vi "Check for Authorization.vi"(8 "error in":errorcluster, 10 "JSON":string, 11 "nats connection in":T1) -> (0 "error out":errorcluster, 2 "dup JSON":string, 3 "dup nats connection":T1)   [LabVIEW 2013, in "NATS Core.lvlib"]
doc: "Check if the server is requesting some form of authorization. If so, verify the client has provided some form of authorization regardless of validity."
uses:
  NATS Core.lvlib
  Controls/nats connection.ctl
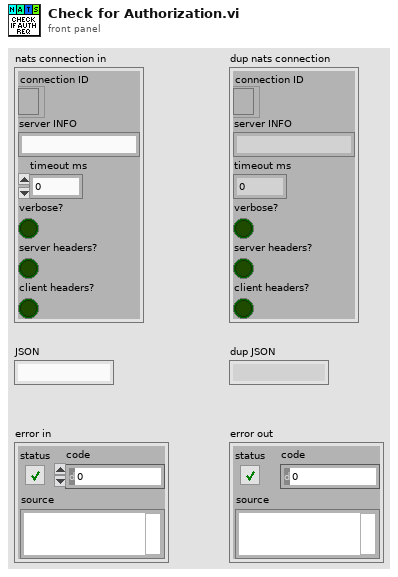
[diagram p1: front panel]
types:
  T1 = typedef "NATS Core.lvlib/nats connection.ctl" = cluster{"connection ID":refnum<k5>, "server INFO":string, "timeout ms":i32, "verbose?":bool, "server headers?":bool, "client headers?":bool}
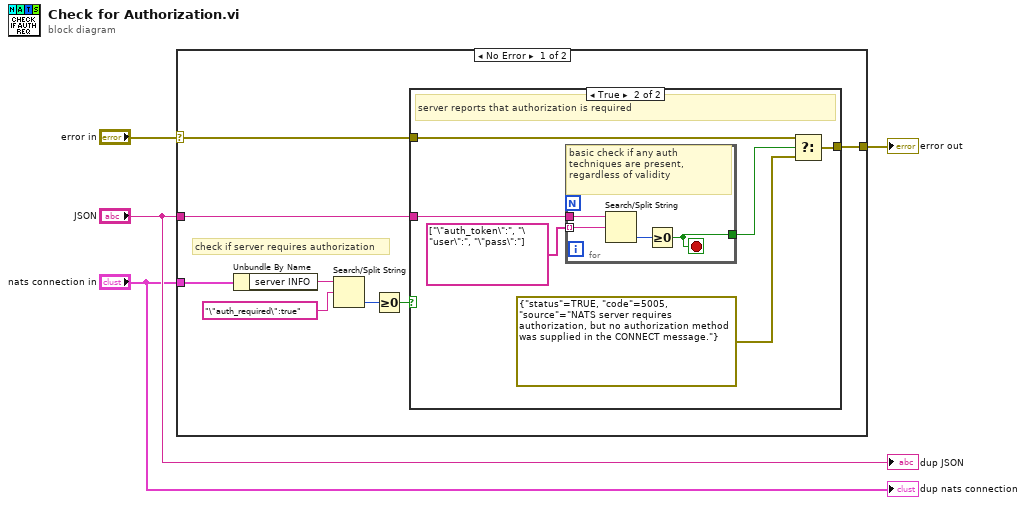
[diagram p0: block diagram]
diagram:
  n1 = case shown="No Error" "error in" {
    selector: "error in" -> [w10 w24]
    tunnel: "JSON" -> [w12 _]
    tunnel: [w11 w24] -> w3
    tunnel: "nats connection in" -> [w5 _]
    frame No Error {
      # "check if server requires authorization"
      n2 = Unbundle By Name(w5) -> ("server INFO"=w8:string)
      n3 = Search/Split String(string=w8, search string/char (-)="\"auth_required\":true") -> (offset of match=w6:i32)  [unwired: 1 in, 2 out]
      n4 = Greater Or Equal To 0?(x=w6) -> (x >= 0?=w9:bool)
      n5 = case shown="True" w9 {
        tunnel: w12 -> [_ w18]
        tunnel: w10 -> [w13 w16]
        tunnel: [w13 w15] -> w11
        frame False {
          # "no server requirement for authorization"
        }
        frame True {
          # "server reports that authorization is required"
          n6 = for {
            tunnel: string[] ["\"auth_token\":", "\"user\":", "\"pass\":"] ("delimiters (\\s,\\t,\\r,\\n)") -> [w23] mode=indexing
            tunnel: w18 -> [w22]
            tunnel: [w20] -> w17
            stop <- w20 stop-if-true
            # "basic check if any auth techniques are present, regardless of validity"
            n7 = Search/Split String(string=w22, search string/char (-)=w23) -> (offset of match=w21:i32)  [unwired: 1 in, 2 out]
            n8 = Greater Or Equal To 0?(x=w21) -> (x >= 0?=w20:bool)
          }
          n9 = Select(t=w16, s=w17, f=errorcluster {"status"=TRUE, "code"=5005, "source"="NATS server requires authorization, but no authorization method was supplied in the CONNECT message."} ("error constant")) -> (s? t:f=w15:errorcluster)
        }
      }
    }
    frame Error {
    }
  }
  "error out" <- w3
  "dup JSON" <- "JSON"
  "dup nats connection" <- "nats connection in"
